vi "Align Tab Control.vi"(8 "error in (no error)":errorcluster, 11 "TabCtl Refnum In":refnum<vi>) -> (0 "error out":errorcluster)   [LabVIEW 2013, in "DCAF UI Elements.lvlib"]
uses:
  Controls/DCAF UI Elements.lvlib
  <vilib>/Utility/miscctls.llb/LVPositionTypeDef.ctl
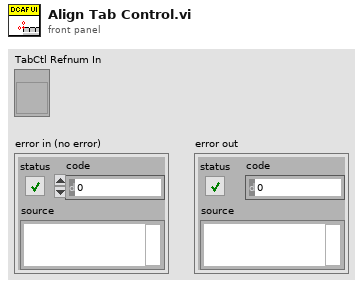
[diagram p1: front panel]
types:
  T1 = typedef "LVPositionTypeDef.ctl" = cluster{"Left":i32, "Top":i32}
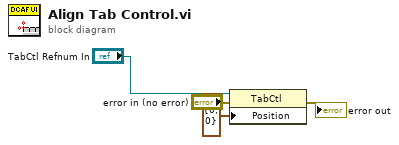
[diagram p0: block diagram]
diagram:
  n1 = property class="TabCtl"(reference="TabCtl Refnum In", error in="error in (no error)", "Position"=T1 {"Left"=0, "Top"=0}) -> (error out=→"error out":errorcluster)  [unwired: 1 out]
